vi "Get VI Ref.vi"(8 "error in (no error)":errorcluster, 10 "Module Names":string[](array[string])) -> (0 "error out":errorcluster, 2 "All Module Ref":refnum<vi>[](array[refnum]))   [LabVIEW 2020]
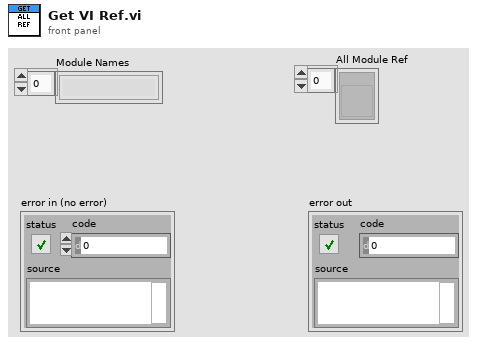
[diagram p1: front panel]
types:
  T1 = enum32{"invalid app kind", "Development System", "Run Time System", "Student Edition", "Embedded LabVIEW", "Evaluation", "Custom"}
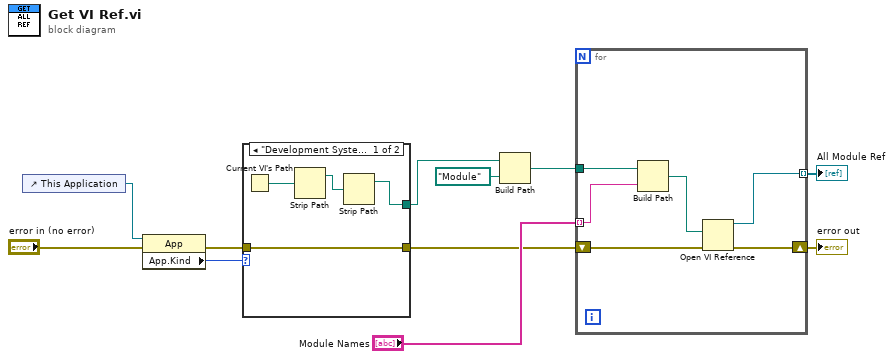
[diagram p0: block diagram]
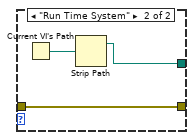
[diagram p2: hidden frame]
diagram:
  n1 = control-ref of="This Application"() -> (w11:refnum<vi>)
  n2 = property class="App"(reference=w11, error in="error in (no error)") -> (error out=w8:errorcluster, "App.Kind"=w9:T1)  [unwired: 1 out]
  n3 = case shown="\"Development System\", Default" w9 {
    tunnel: w8 -> [w13 w16]
    tunnel: [w13 w16] -> w3
    tunnel: [w12 w17] -> w7
    frame "Development System", Default {
      n4 = Current VI's Path() -> (path=w15:path)
      n5 = Strip Path(path=w15) -> (stripped path=w14:path)  [unwired: 1 out]
      n6 = Strip Path(path=w14) -> (stripped path=w12:path)  [unwired: 1 out]
    }
    frame "Run Time System" {
      n7 = Current VI's Path() -> (path=w18:path)
      n8 = Strip Path(path=w18) -> (stripped path=w17:path)  [unwired: 1 out]
    }
  }
  n9 = Build Path(base path=w7, name or relative path=path "Module") -> (appended path=w4:path)
  n10 = for {
    tunnel: "Module Names" -> [w23] mode=indexing
    tunnel: w4 -> [w24]
    shift-right: [w20] -> w2
    shift-left: w3 -> [w22]
    tunnel: [w19] -> w1 mode=indexing
    n11 = Build Path(base path=w24, name or relative path=w23) -> (appended path=w21:path)
    n12 = Open VI Reference(vi path=w21, error in (no error)=w22) -> (vi reference=w19:refnum<vi>, error out=w20:errorcluster)  [unwired: 4 in]
  }
  "error out" <- w2
  "All Module Ref" <- w1
